vi "Configure GPIO Routes.vi"(0 "fpga interface in":refnum<k20>, 5 "gpio routes":T1[](array[typedef]) {"Serial Channel" max=3 step=1}, 11 "error in (no error)":errorcluster) -> (4 "fpga interface out":refnum<k20>, 15 "error out":errorcluster)   [LabVIEW 2023, in "GettingStarted_Common_148X_Host.lvlib"]
uses:
  GettingStarted_Common_148X_Host.lvlib
  Types/GPIO Route Configuration.ctl
  Types/GPIO Route Direction.ctl
  Types/GPIO Route Line.ctl
  Types/148x_Common_FPGA_Reference.ctl
  <vilib>/Utility/error.llb/Error Cluster From Error Code.vi
  <vilib>/rvi/errors/niLvFpgaAdjustHostInterfaceError.vi
  <vilib>/rvi/interface/nirviReadWriteControl/nirviReadWriteControl.xnode
  NiFpgaLv.dll
  <vilib>/rvi/interface/Simulation/niFpgaSimulationCallBeginRW.vi
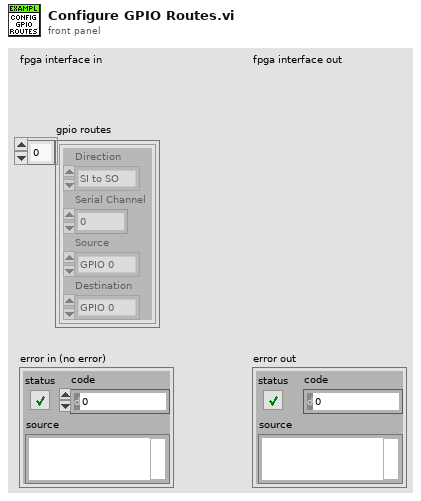
[diagram p1: front panel]
types:
  T1 = typedef "GettingStarted_Common_148X_Host.lvlib/GPIO Route Configuration.ctl" = cluster{"Direction":T2, "Serial Channel":u8, "Source":T3, "Destination":T3}
  T2 = typedef "GettingStarted_Common_148X_Host.lvlib/GPIO Route Direction.ctl" = enum8{"SO to SI", "SI to SO"}
  T3 = typedef "GettingStarted_Common_148X_Host.lvlib/GPIO Route Line.ctl" = enum16{"GPIO 0", "GPIO 1", "GPIO 2", "GPIO 3", "GPIO 4", "GPIO 5", "GPIO 6", "GPIO 7", "GPIO 8", "GPIO 9", "GPIO 10", "User"}
  T4 = typedef "GettingStarted_Common_148X_Host.lvlib/148x_Common_FPGA_Reference.ctl" = refnum<k20>
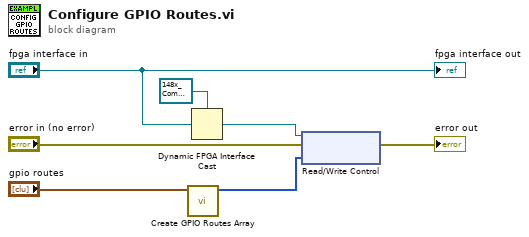
[diagram p0: block diagram]
diagram:
  n1 = call "Create GPIO Routes Array.vi"("gpio route configurations"="gpio routes") -> ("gpio routes"=w2:i8[])  [unwired: 10 in]
  n2 = Dynamic FPGA Interface Cast(Session In=T4 refnum ("Type"), Type="fpga interface in") -> (Session Out=w4:T4)
  n3 = xnode "Read/Write Control"("FPGA VI Reference In"=w4, "error in"="error in (no error)", "gpio routes"=w2) -> ("error out"=→"error out":errorcluster)  [unwired: 1 out]
  "fpga interface out" <- "fpga interface in"
